vi "writeToXML.vi"(8 "error in (no error)":errorcluster, 10 "ClassLabel":string, 11 "DifftrackAzEl in":refnum<class "DifftrackAzEl.lvclass">) -> (0 "error out":errorcluster, 2 "XML out":string, 3 "DifftrackAzEl out":refnum<class "DifftrackAzEl.lvclass">)   [LabVIEW 2022 SP3, in "TCSDataDefinitions.lvlib" / "TCSCommand.lvlib" / "TargetConfiguration.lvlib" / "Target.lvlib" / "DifftrackAzEl.lvclass"]
uses:
  DifftrackAzEl.lvclass
  <userlib>/Common/UnitsAndXML/FlattenItemWithUnitToXML/FlattenAngularVelocityToXML/AngularVelocityUnit.ctl
  DifftrackAzEl.lvclass/DifftrackAzEl.ctl
  Difftrack.lvclass
  <userlib>/Common/UnitsAndXML/UnitsAndXML.lvlib
  <userlib>/Common/XML/XMLGenerator/XMLGenerator.lvclass
  <userlib>/Common/XML/XMLAttributeGenerator/XMLAttributeGenerator.lvclass
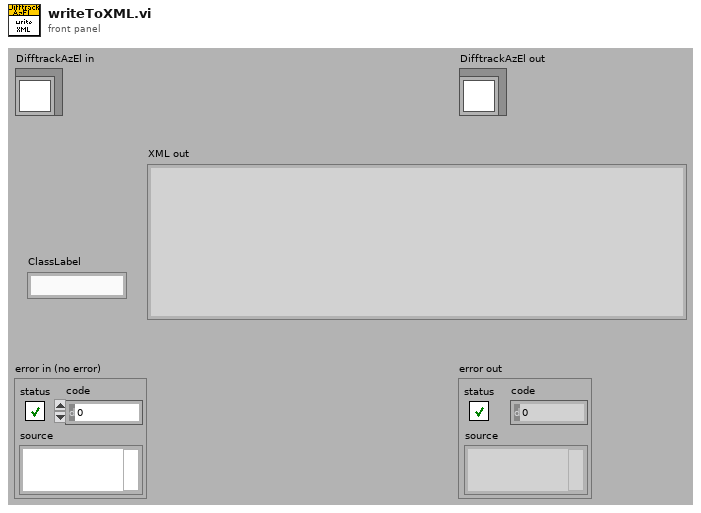
[diagram p1: front panel]
types:
  T1 = typedef "UnitsAndXML.lvlib/AngularVelocityUnit.ctl" = enum16{"\"/a", "deg/s", "\"/s"}
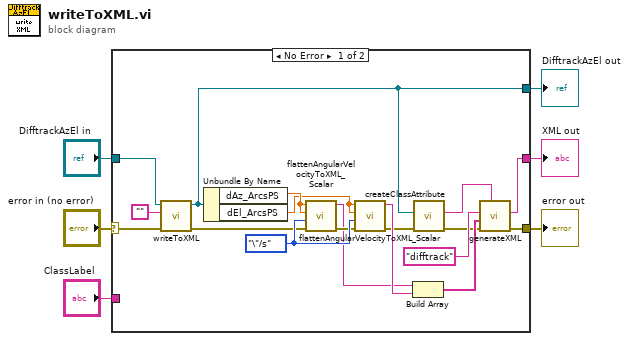
[diagram p0: block diagram]
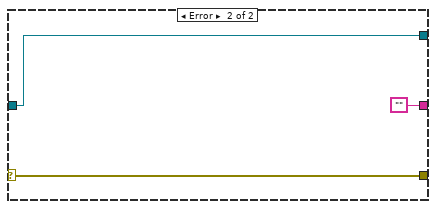
[diagram p2: hidden frame]
diagram:
  n1 = case shown="No Error" "error in (no error)" {
    selector: "error in (no error)" -> [w17 w27]
    tunnel: [w16 w27] -> w5
    tunnel: [w10 w26] -> w3
    tunnel: "DifftrackAzEl in" -> [w23 w26]
    tunnel: [w11 ""] -> w2
    tunnel: "ClassLabel" -> [_ _]
    frame No Error {
      w21 = AngularVelocityUnit."\"/s" ("angularVelocityUnitInXML")
      n2 = call-parent "writeToXML.vi"("error in (no error)"=w17, "ClassLabel"="", "Difftrack in"=w23) -> ("error out"=w18:errorcluster, "Difftrack out"=w10:refnum<class "DifftrackAzEl.lvclass">)  [unwired: 6 in, 1 out]
      n3 = Unbundle By Name(w10) -> ("dAz_ArcsPS"=w22:dbl[unit], "dEl_ArcsPS"=w20:dbl[unit])
      n4 = call <userlib>:"flattenAngularVelocityToXML_Scalar.vi"("error in (no error)"=w18, "angularVelocityUnitInXML"=w21, "anuglarVelocityAgain"=w22, "angularVelocity"=w22) -> ("error out"=w19:errorcluster, "xmlString"=w14:string)  [unwired: 6 in]
      n5 = call <userlib>:"flattenAngularVelocityToXML_Scalar.vi"("error in (no error)"=w19, "angularVelocityUnitInXML"=w21, "anuglarVelocityAgain"=w20, "angularVelocity"=w20) -> ("error out"=w9:errorcluster, "xmlString"=w15:string)  [unwired: 6 in]
      n6 = Build Array(w14, w15) -> (w13:string[])
      n7 = call <userlib>:"createClassAttribute.vi"("error in (no error)"=w9, "LVClass In"=w10) -> ("error out"=w8:errorcluster, "AttributeString"=w7:string)  [unwired: 7 in, 1 out]
      n8 = call <userlib>:"generateXML.vi"("attributeString"=w7, "error in"=w8, "childrenXML"=w13, "elementName"="difftrack" ("Class Label")) -> ("error out"=w16:errorcluster, "XML out"=w11:string)  [unwired: 5 in, 1 out]
    }
    frame Error {
    }
  }
  "error out" <- w5
  "DifftrackAzEl out" <- w3
  "XML out" <- w2
